vi "LAKESHORE_10_01_2023.vi"() -> ()   [LabVIEW 2020]
panel:
  in  "Channel":T1(ring)
  in  "Average Number of readings \nper iterations":i64
  in  "Select Parameter":enum16{"Resistance(ohms)", "Temperature(K)"}(ring)
  out "XY Graph":cluster{"X":dbl[], "Y":dbl[]}[](graph)
  out "Measured Average Value":dbl
  in  "VISA resource name":refnum<visa-resource-name>
  # "LAKE SHORE"
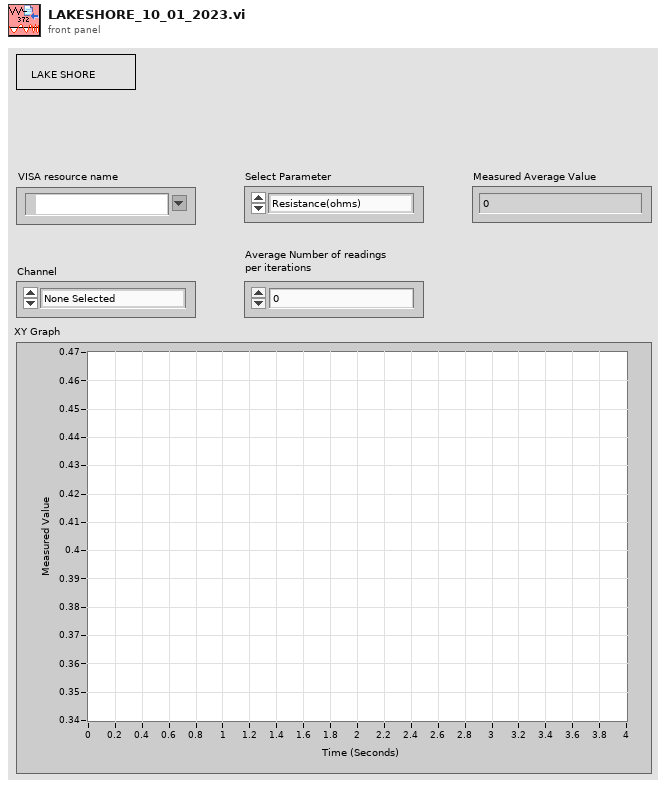
[diagram p1: front panel]
types:
  T1 = enum16{"None Selected", "1", "2", "3", "4", "5", "6", "7", "8", "9", "10", "11", "12", "13", "14", "15", "16"}
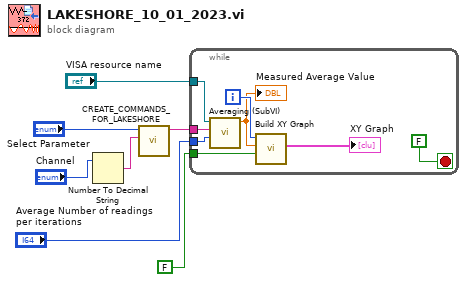
[diagram p0: block diagram]
diagram:
  n1 = Number To Decimal String(number="Channel") -> (decimal integer string=w2:string)  [unwired: 1 in]
  n2 = call "CREATE_COMMANDS_FOR_LAKESHORE.vi"("Channel"=w2, "Select Parameter"="Select Parameter") -> ("result string"=w6:string)  [unwired: 9 in]
  n3 = while {
    tunnel: "VISA resource name" -> [w10]
    tunnel: w6 -> [w11]
    tunnel: FALSE ("Reset") -> [w12]
    tunnel: "Average Number of readings \nper iterations" -> [w8]
    i -> [w13]
    stop <- FALSE stop-if-true
    n4 = call "Averaging (SubVI).vi"("N"=w8, "result string"=w11, "VISA Refnum in"=w10) -> ("Numeric"=w9:dbl)  [unwired: 8 in]
    "Measured Average Value" <- w9
    n5 = call "Build XY Graph"("Reset"=w12, "Y Input"=w9, "X Input"=w13) -> ("XY Graph"=→"XY Graph":cluster{"X":dbl[], "Y":dbl[]}[])  [unwired: 7 in, 1 out]
  }
